vi "determineClassVersion.vi"(8 "error in (no error)":errorcluster, 10 "className":string) -> (0 "error out":errorcluster, 2 "Version":T1)   [LabVIEW 2020, in "JKI JSON Object Serialization.lvlib" / "OOP_Utility.lvlib" / "Reflection.lvclass"]
doc: "Given a class name, determine the version number of the input object. Version Number is formatted as a byte array.\n\nGCraftsman JSON Object Serialization Toolkit\nwww.GCraftsman.com\nCopyright (c) 2017, GCraftsman"
uses:
  Reflection.lvclass
  Reflection.lvclass/Reflection.ctl
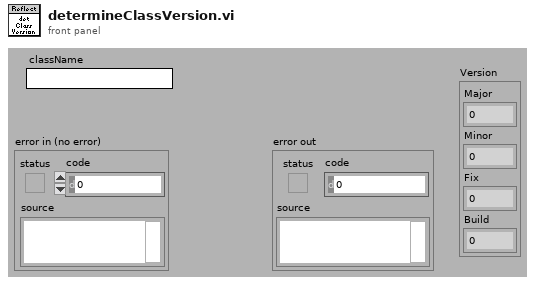
[diagram p1: front panel]
types:
  T1 = cluster{"Major":u16, "Minor":u16, "Fix":u16, "Build":u16}
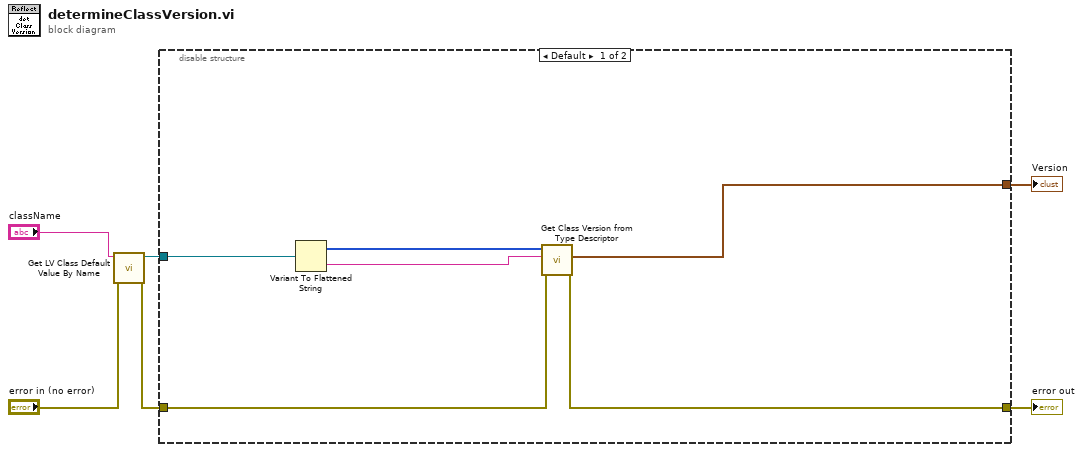
[diagram p0: block diagram]
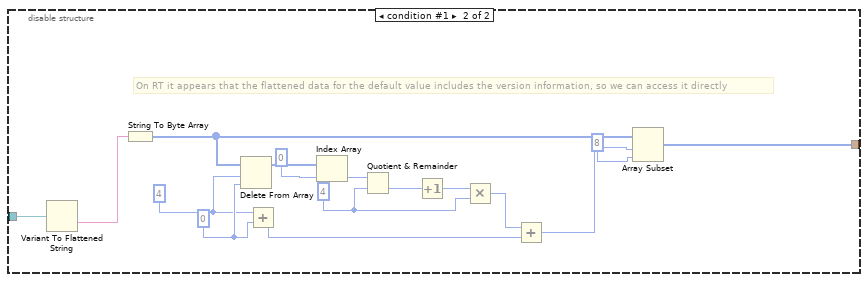
[diagram p2: hidden frame]
diagram:
  n1 = call <vilib>:"Get LV Class Default Value By Name.vi"("error in (no error)"="error in (no error)", "class name"="className") -> ("error out"=w2:errorcluster, "object"=w5:refnum<class>)  [unwired: 8 in]
  n2 = disable-structure shown="Default" {
    disable-tunnel: [w7 w27] -> w6
    disable-tunnel: w5 -> [w10 w26]
    disable-tunnel: w2 -> [w9 _]
    disable-tunnel: [w8 _] -> w1
    frame condition #0 (active) {
      n3 = Variant To Flattened String(Variant=w10) -> (data string=w12:string, 1:w11:i16[])
      n4 = call "Get Class Version from Type Descriptor.vi"("error in"=w9, "data string"=w12, "type string"=w11) -> ("error out"=w8:errorcluster, "Version"=w7:T1)  [unwired: 7 in]
    }
    frame condition #1 {
      w21 = u8 4 ("y")
      w14 = 0 ("index")
      w13 = 4 ("offset (0)")
      # "On RT it appears that the flattened data for the default value includes the version information, so we can access it directly"
      n5 = Variant To Flattened String(Variant=w26) -> (data string=w15:string)  [unwired: 1 out]
      n6 = String To Byte Array(string=w15) -> (unsigned byte array=w17:u8[])
      n7 = Delete From Array(array=w17, length=w13, index=w14) -> (array with subset deleted=w19:u8[])  [unwired: 1 out]
      n8 = Add(x=w13, y=w14) -> (x+y=w16:i32)
      n9 = Index Array(array=w19, index=0) -> (element=w24:u8)
      n10 = Quotient & Remainder(x=w24, y=w21) -> (floor(x/y)=w23:u8)  [unwired: 1 out]
      n11 = Increment(x=w23) -> (x+1=w22:u8)
      n12 = Multiply(x=w22, y=w21) -> (x*y=w20:u8)
      n13 = Add(x=w20, y=w16) -> (x+y=w18:i32)
      n14 = Array Subset(array=w17, index=w18, length=8) -> (w27:u8[])
    }
  }
  "Version" <- w6
  "error out" <- w1
